vi "time_array.vi"() -> ()   [LabVIEW 2017]
panel:
  out "Output":dbl[][](array[numeric])
  out "real time":dbl[](array[numeric])
  out "Waveform Chart":dbl(graph)
  out "day":dbl(knob) scale=0.0..10.0
  out "hr":dbl(knob) scale=0.0..10.0
  out "min":dbl(knob) scale=0.0..60.0
  out "ii":i32
  in  "stop":bool
  out "s":dbl(knob) scale=0.0..60.0
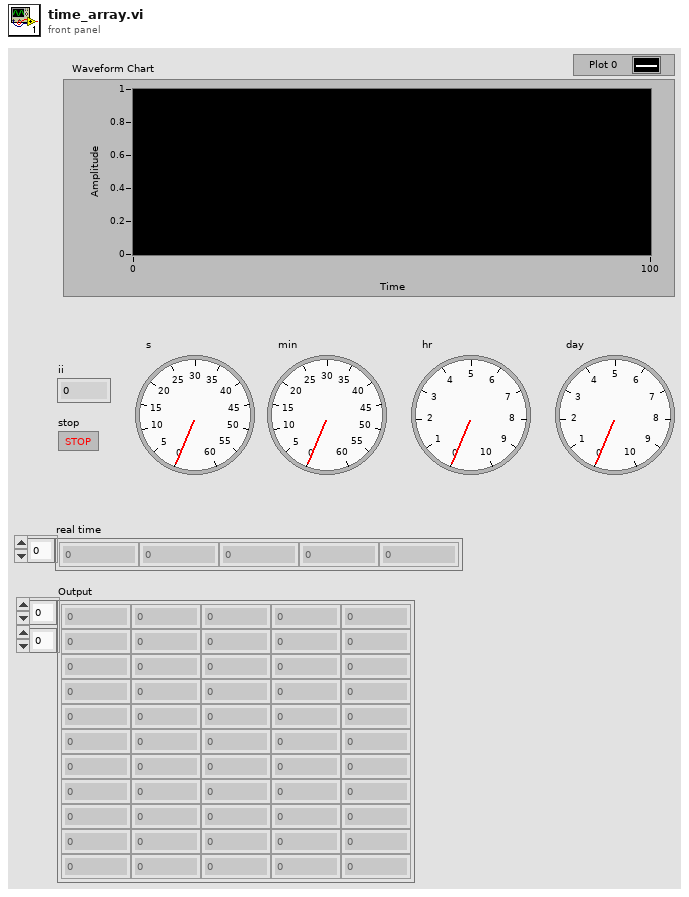
[diagram p1: front panel]
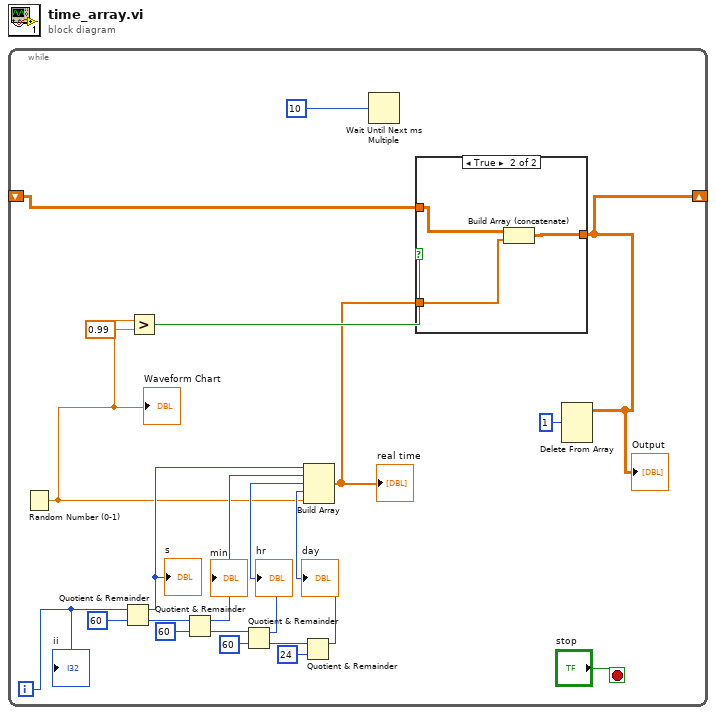
[diagram p0: block diagram]
diagram:
  n1 = while {
    shift-right: [w2] -> _
    shift-left: _ -> [w3]
    i -> [w19]
    stop <- "stop" stop-if-true
    n2 = Random Number (0-1)() -> (number: 0 to 1=w6:dbl)
    "Waveform Chart" <- w6
    n3 = Quotient & Remainder(x=w19, y=60) -> (x-y*floor(x/y)=w10:i32, floor(x/y)=w17:i32)
    "s" <- w10
    n4 = Greater?(x=w6, y=0.99) -> (0:w5:bool)
    n5 = Quotient & Remainder(x=w17, y=60) -> (x-y*floor(x/y)=w9:i32, floor(x/y)=w15:i32)
    "min" <- w9
    n6 = Quotient & Remainder(x=w15, y=60) -> (x-y*floor(x/y)=w8:i32, floor(x/y)=w13:i32)
    "hr" <- w8
    n7 = Quotient & Remainder(x=w13, y=24) -> (x-y*floor(x/y)=w7:i32)  [unwired: 1 out]
    "day" <- w7
    n8 = Build Array(w10, w9, w8, w7, w6) -> (w4:dbl[])
    "real time" <- w4
    n9 = Wait Until Next ms Multiple(millisecond multiple=10) -> ()  [unwired: 1 out]
    n10 = case shown="True" w5 {
      tunnel: w4 -> [_ w24]
      tunnel: w3 -> [w22 w25]
      tunnel: [w22 w23] -> w2
      frame False {
      }
      frame True {
        n11 = Build Array (concatenate)(w25, w24) -> (w23:dbl[][])
      }
    }
    "Output" <- w2
    n12 = Delete From Array(array=w2, length=1) -> ()  [unwired: 2 in, 2 out]
    "ii" <- w19
  }
